vi "Elevator Controller.vi"(8 "error in (no error)":errorcluster, 9 "Notify when settled?":bool, 10 "State in":T2=enum."Tote 3", 11 "Elevator Inputs":T1={"Up"=FALSE, "Down"=FALSE, "Bin Modifier"=FALSE, "Pickup"=FALSE, "Top LS"=FALSE, "Bottom LS"=FALSE, "Encoder Position"=-2958.0, "Encoder Velocity"=0.0, "Manual Control"=-0.0}) -> (0 "error out":errorcluster, 1 "Settled?":bool=TRUE, 2 "Output":dbl=0.0975, 3 "State out":T2=enum."Tote 3")   [LabVIEW 2014]
uses:
  Elevator States.ctl
  Elevator Input Data.ctl
  Elevator Control Mode.ctl
  Utilities/Sensor Refname.ctl
  Elevator Direction.ctl
  <vilib>/Rock Robotics/Network Tables/SD Read Boolean.vi
  Robot Global Data.vi
  Utilities/Sensor Refname to String.vi
  <vilib>/Rock Robotics/Network Tables/SD Write Number.vi
  <vilib>/addons/control/pid/pid.llb/PID Advanced (DBL).vi
  <vilib>/addons/control/pid/NI_PID_pid.lvlib
panel:
  in  "Tab Control":enum32{"Inputs", "Outputs", "PID", "Config"}(tab)=enum."PID"
  in  "PID gains":T3={"proportional gain (Kc)"=-0.0025, "integral time (Ti, min)"=0.0, "derivative time (Td, min)"=0.0} {"derivative time (Td, min)" format="%.3f"; "integral time (Ti, min)" format="%.3f"; "proportional gain (Kc)" format="%.3f"}
  in  "PID output range":cluster{"output high":dbl, "output low":dbl}={"output high"=1.0, "output low"=-0.75} {"output low" format="%.2f"; "output high" format="%.2f"}
  in  "Setpoint range":cluster{"setpoint high":dbl, "setpoint low":dbl}={"setpoint high"=100.0, "setpoint low"=-6000.0} {"setpoint high" format="%.2f"; "setpoint low" format="%.2f"}
  in  "reinitialize? (F)":bool
  in  "Deadzone":dbl=0.15
  in  "Setpoint Diff":dbl=250.0
  in  "Motor Diff":dbl=2.0
  in  "Enable motor ramping?":bool
  in  "Enable setpoint chasing?":bool=TRUE
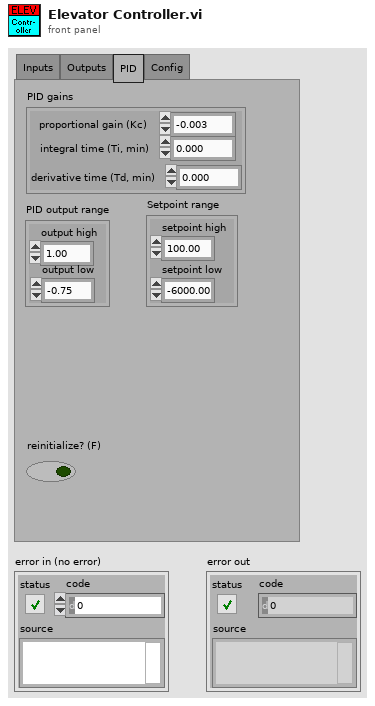
[diagram p1: front panel]
types:
  T1 = typedef "Elevator Input Data.ctl" = cluster{"Up":bool, "Down":bool, "Bin Modifier":bool, "Pickup":bool, "Top LS":bool, "Bottom LS":bool, "Encoder Position":dbl, "Encoder Velocity":dbl, "Manual Control":dbl}
  T2 = typedef "Elevator States.ctl" = enum16{"Ground", "Tote 1", "Tote 2", "Tote 3", "Tote 4", "Tote 5", "Tote 6"}
  T3 = cluster{"proportional gain (Kc)":dbl, "integral time (Ti, min)":dbl, "derivative time (Td, min)":dbl}
  T4 = typedef "Elevator Control Mode.ctl" = enum16{"PID", "PID to Manual", "Manual", "Manual to PID"}
  T5 = typedef "Sensor Refname.ctl" = enum16{"Gyro", "Elevator Top LS", "Elevator Bottom LS", "Claw Outside LS", "Left Drive Encoder", "Right Drive Encoder", "Strafe Encoder", "Elevator Encoder", "Ultrasonic Forward", "Ultrasonic Back", "Arm Angle POT", "Arm Clapper POT", "Accelerometer", "Tote LS", "DIP 1", "DIP 2", "DIP 3", "DIP 4"}
  T6 = typedef "Elevator Direction.ctl" = enum16{"Up", "Down"}
  T7 = typedef "WPI_PotentiometerDevRef.ctl" = cluster{"DevStatus":errorcluster, "Controller":T8, "Analog Channel":T9, "Invert Output":bool}
  T8 = typedef "FPGA_TypedefAnalogModule.ctl" = enum16{"Controller 1"}
  T9 = typedef "FPGA_AIChannel.ctl" = enum8{"AI 0", "AI 1", "AI 2", "AI 3", "AI MXP 0", "AI MXP 1", "AI MXP 2", "AI MXP 3", "Invalid"}
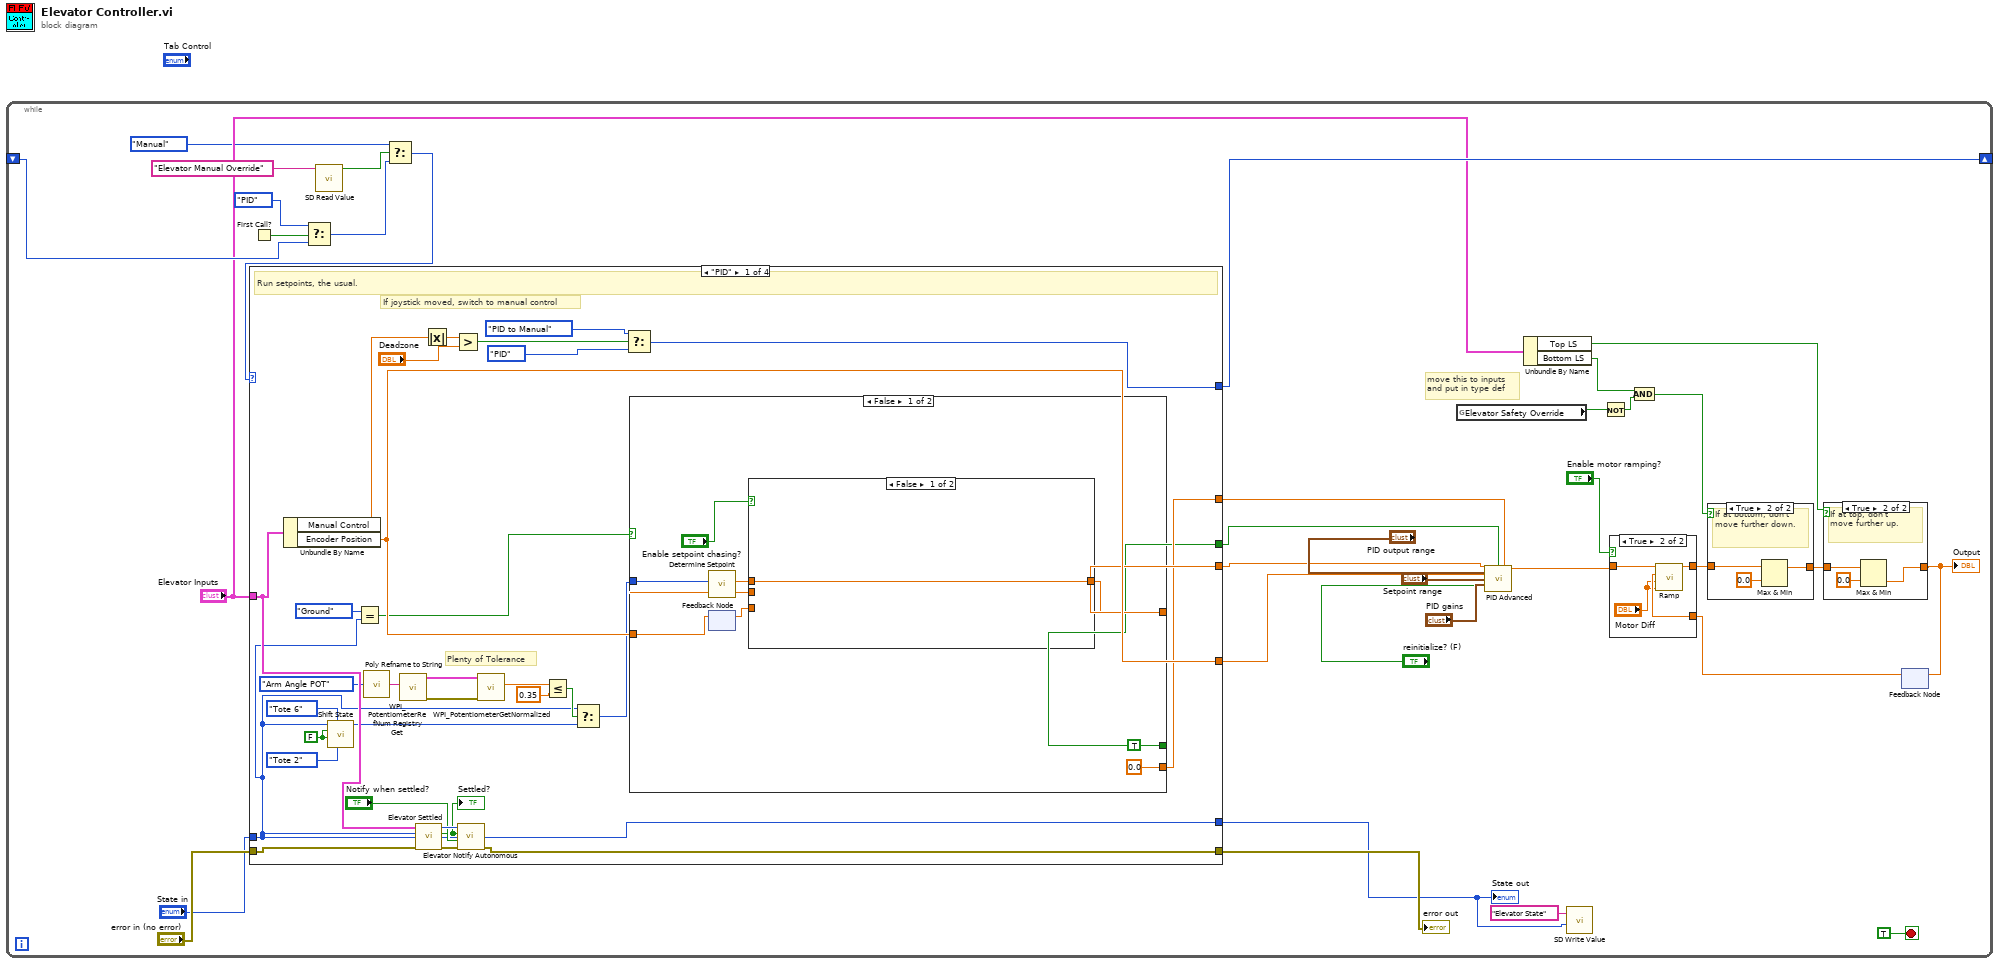
[diagram p0: block diagram]
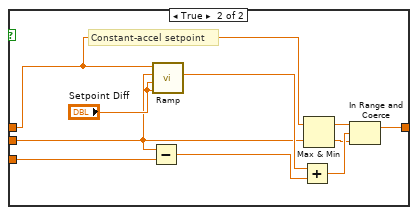
[diagram p5: hidden frame]
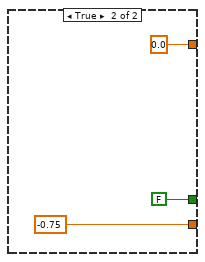
[diagram p6: hidden frame]
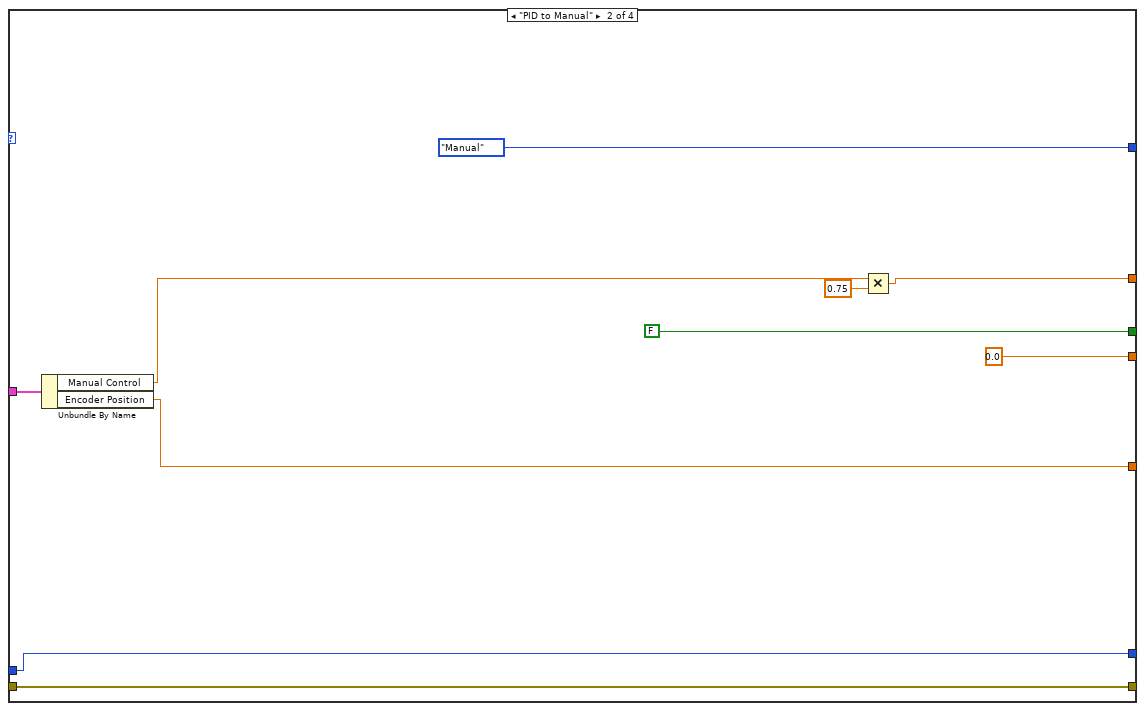
[diagram p7: hidden frame]
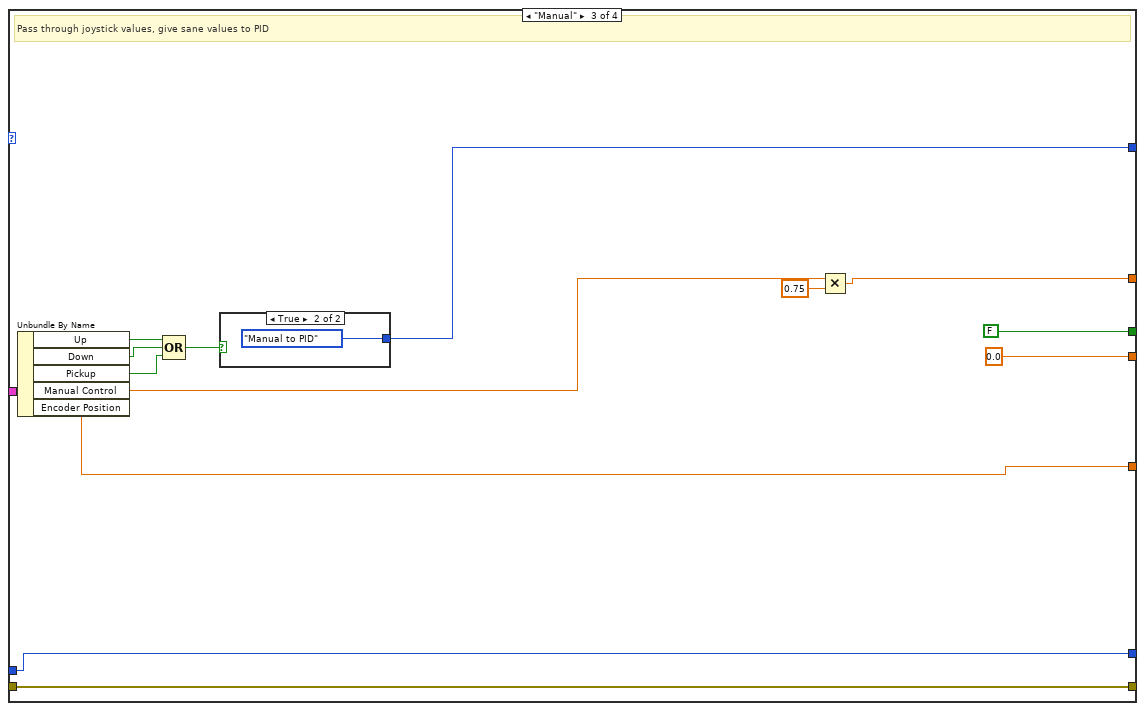
[diagram p8: hidden frame]
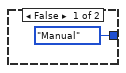
[diagram p9: hidden frame]
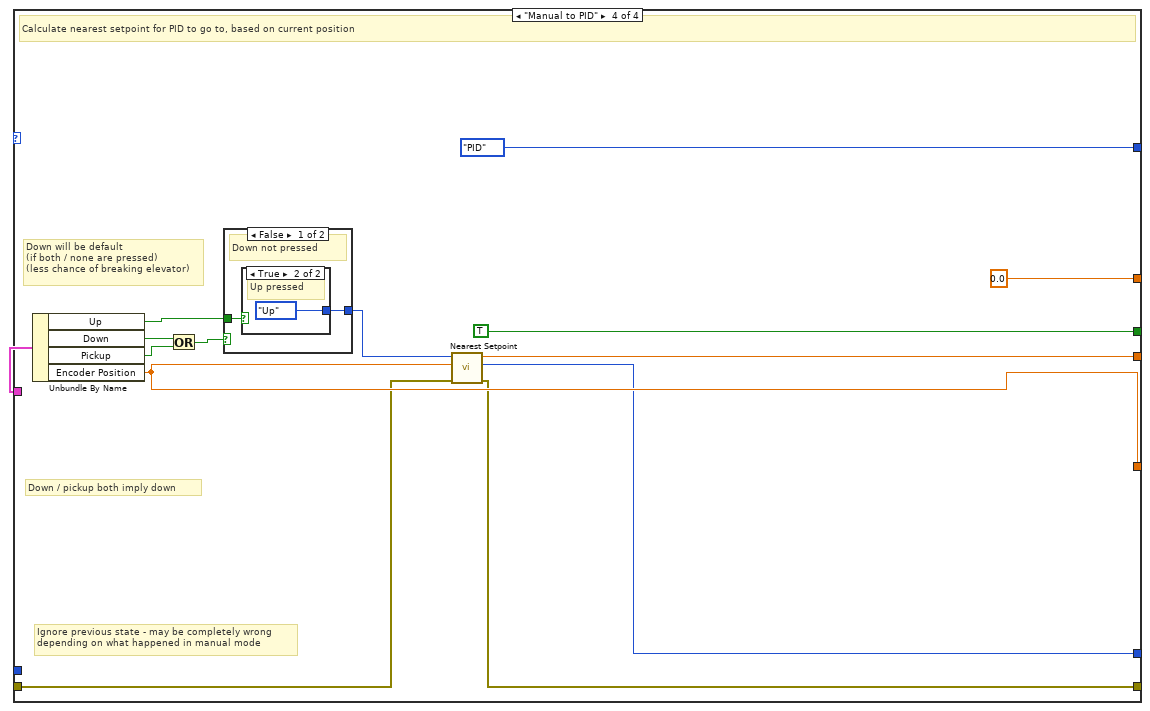
[diagram p10: hidden frame]
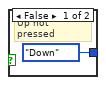
[diagram p11: hidden frame]
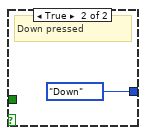
[diagram p12: hidden frame]
diagram:
  n1 = while {
    shift-right: [w33] -> _
    shift-left: _ -> [w35]
    stop <- TRUE stop-if-true
    # "move this to inputs \nand put in type def"
    n2 = First Call?() -> (First Call?: T/F=w5:bool)
    n3 = Select(t=Elevator_Control_Mode."PID", s=w5, f=w35) -> (s? t:f=w12:T4)
    n4 = call-poly <vilib>:"SD Read Value.vi"("Name"="Elevator Manual Override") -> ("Boolean"=w9:bool)  [unwired: 8 in, 2 out]
    n5 = Select(t=Elevator_Control_Mode."Manual", s=w9, f=w12) -> (s? t:f=w11:T4)
    n6 = case shown="\"PID\"" w11 {
      tunnel: "Elevator Inputs" -> [w77 w111 w127 w143]
      tunnel: [w66 0.0 ("Setpoint") 0.0 ("Manual Control") w137] -> w15
      tunnel: [w62 FALSE FALSE TRUE] -> w25
      tunnel: [w72 Elevator_Control_Mode."Manual" w121 Elevator_Control_Mode."PID"] -> w33
      tunnel: [w67 w110 w118 w134] -> w28
      tunnel: [w65 w105 w115 0.0 ("Manual Control")] -> w24
      tunnel: [w53 w107 w117 w132] -> w6
      tunnel: "State in" -> [w53 w107 w117 _]
      tunnel: "error in (no error)" -> [w71 w106 w116 w130]
      tunnel: [w70 w106 w116 w131] -> w21
      frame "PID" {
        w50 = FALSE
        # "Plenty of Tolerance"
        # "If joystick moved, switch to manual control"
        # "Run setpoints, the usual."
        n7 = Unbundle By Name(w77) -> ("Manual Control"=w74:dbl, "Encoder Position"=w67:dbl)
        n8 = call "Shift State.vi"("Lower bound"=Elevator_States."Tote 2" ("x"), "Upper bound"=Elevator_States."Tote 6" ("x"), "Decrement"=w50, "Increment"=w50, "State in"=w53) -> ("State out"=w49:i32)  [unwired: 6 in]
        n9 = Equal?(x=Elevator_States."Ground", y=w53) -> (x = y?=w64:bool)
        n10 = call-poly "Poly Refname to String.vi"("Sensor Refnames"=Sensor_Refname."Arm Angle POT" ("Sensor Refname")) -> ("Refname"=w60:string)
        n11 = call <vilib>:"WPI_PotentiometerRefNum Registry Get.vi"("refnum name"=w60) -> ("error out"=w58:errorcluster, "PotDevRef"=w59:T7)  [unwired: 9 in]
        n12 = call "Elevator Settled.vi"("error in (no error)"=w71, "State"=w53, "Elevator Inputs"=w77) -> ("error out"=w79:errorcluster, "Settled?"=w78:bool, "State"=w81:T2)  [unwired: 6 in]
        "Settled?" <- w78
        n13 = Absolute Value(x=w74) -> (abs(x)=w76:dbl)
        n14 = Greater?(x=w76, y="Deadzone") -> (0:w73:bool)
        n15 = call "Elevator Notify Autonomous.vi"("error in (no error)"=w79, "Notify when settled?"="Notify when settled?", "Settled?"=w78, "State"=w81) -> ("error out"=w70:errorcluster)  [unwired: 7 in]
        n16 = call <vilib>:"WPI_PotentiometerGetNormalized.vi"("error in"=w58, "PotDevRef"=w59) -> ("Normalized Value"=w57:dbl)  [unwired: 7 in, 2 out]
        n17 = Less Or Equal?(x=w57, y=0.35) -> (x <= y?=w55:bool)
        n18 = Select(t=w53, s=w55, f=w49) -> (s? t:f=w54:i32)
        n19 = Select(t=Elevator_Control_Mode."PID to Manual", s=w73, f=Elevator_Control_Mode."PID" ("t")) -> (s? t:f=w72:T4)
        n20 = case shown="False" w64 {
          tunnel: [TRUE FALSE] -> w62
          tunnel: w54 -> [w84 _]
          tunnel: [w87 0.0 ("Setpoint")] -> w66
          tunnel: w67 -> [w83 _]
          tunnel: [0.0 ("Manual Control") -0.75 ("Manual Control")] -> w65
          frame False {
            n21 = call "Determine Setpoint.vi"("Elevator State"=w84) -> ("Setpoint"=w85:dbl)  [unwired: 9 in, 1 out]
            n22 = feedback #1() -> (w82:dbl)  [unwired: 1 in]
            n23 = feedback-in #1(w83) -> ()
            n24 = case shown="False" "Enable setpoint chasing?" {
              tunnel: w85 -> [w90 w95]
              tunnel: [w90 w91] -> w87
              tunnel: w83 -> [_ w94]
              tunnel: w82 -> [_ w99]
              frame False {
              }
              frame True {
                # "Constant-accel setpoint"
                n25 = Subtract(x=w94, y=w99) -> (x-y=w97:dbl)
                n26 = call "Ramp.vi"("Negative Change"="Setpoint Diff", "Positive Change"="Setpoint Diff", "Prev Motor"=w94, "Input"=w95) -> ("Motor Output"=w100:dbl)  [unwired: 6 in, 1 out]
                n27 = Add(x=w100, y=w97) -> (x+y=w96:dbl)
                n28 = Max & Min(x=w95, y=w94) -> (max(x,y)=w93:dbl, min(x,y)=w92:dbl)
                n29 = In Range and Coerce(upper limit=w93, x=w96, lower limit=w92) -> (coerced(x)=w91:dbl)  [unwired: 1 out]
              }
            }
          }
          frame True {
          }
        }
      }
      frame "PID to Manual" {
        n30 = Unbundle By Name(w111) -> ("Manual Control"=w109:dbl, "Encoder Position"=w110:dbl)
        n31 = Multiply(x=w109, y=0.75) -> (x*y=w105:dbl)
      }
      frame "Manual" {
        # "Pass through joystick values, give sane values to PID"
        n32 = Unbundle By Name(w127) -> ("Up"=w125:bool, "Down"=w124:bool, "Pickup"=w123:bool, "Manual Control"=w120:dbl, "Encoder Position"=w118:dbl)
        n33 = Compound Arithmetic op=OR(w125, w124, w123) -> (w122:bool)
        n34 = case shown="True" w122 {
          tunnel: [Elevator_Control_Mode."Manual" Elevator_Control_Mode."Manual to PID"] -> w121
          frame False {
          }
          frame True {
          }
        }
        n35 = Multiply(x=w120, y=0.75) -> (x*y=w115:dbl)
      }
      frame "Manual to PID" {
        # "Ignore previous state - may be completely wrong\ndepending on what happened in manual mode"
        # "Down / pickup both imply down"
        # "Down will be default\n(if both / none are pressed)\n(less chance of breaking elevator)"
        # "Calculate nearest setpoint for PID to go to, based on current position"
        n36 = Unbundle By Name(w143) -> ("Up"=w139:bool, "Down"=w142:bool, "Pickup"=w141:bool, "Encoder Position"=w134:dbl)
        n37 = Or(x=w142, y=w141) -> (x .or. y?=w140:bool)
        n38 = case shown="False" w140 {
          tunnel: w139 -> [w144 _]
          tunnel: [w145 Elevator_Direction."Down" ("Direction")] -> w138
          frame False {
            # "Down not pressed"
            n39 = case shown="True" w144 {
              tunnel: [Elevator_Direction."Down" ("Direction") Elevator_Direction."Up" ("Direction")] -> w145
              frame False {
                # "Up not pressed"
              }
              frame True {
                # "Up pressed"
              }
            }
          }
          frame True {
            # "Down pressed"
          }
        }
        n40 = call "Nearest Setpoint.vi"("error in (no error)"=w130, "Encoder"=w134, "Direction"=w138) -> ("error out"=w131:errorcluster, "State"=w132:T2, "Setpoint"=w137:dbl)  [unwired: 6 in]
      }
    }
    "State out" <- w6
    "error out" <- w21
    n41 = global read "Robot Global Data.vi" "Elevator Safety Override"() -> (w2:bool)
    n42 = call-poly <vilib>:"PID Advanced.vi"("setpoint"=w15, "output range"="PID output range", "auto? (T)"=w25, "manual control"=w24, "process variable"=w28, "setpoint range"="Setpoint range", "PID gains"="PID gains", "reinitialize? (F)"="reinitialize? (F)") -> ("output"=w20:dbl)  [unwired: 6 in, 1 out]
    n43 = Unbundle By Name("Elevator Inputs") -> ("Top LS"=w31:bool, "Bottom LS"=w4:bool)
    n44 = call-poly <vilib>:"SD Write Value.vi"("Numeric"=w6, "Name"="Elevator State") -> ()  [unwired: 8 in, 2 out]
    n45 = Not(x=w2) -> (.not. x?=w3:bool)
    n46 = And(x=w4, y=w3) -> (x .and. y?=w1:bool)
    n47 = feedback #2() -> (w17:dbl)  [unwired: 1 in]
    n48 = case shown="True" "Enable motor ramping?" {
      tunnel: w20 -> [w36 w40]
      tunnel: [w36 w39] -> w19
      tunnel: w17 -> [_ w38]
      frame False {
      }
      frame True {
        n49 = call "Ramp.vi"("Negative Change"="Motor Diff", "Positive Change"="Motor Diff", "Prev Motor"=w38, "Input"=w40) -> ("Motor Output"=w39:dbl)  [unwired: 6 in, 1 out]
      }
    }
    n50 = case shown="True" w1 {
      tunnel: [w45 w48] -> w32
      tunnel: w19 -> [w45 w46]
      frame False {
      }
      frame True {
        # "If at bottom, don't move further down."
        n51 = Max & Min(x=w46, y=0.0 ("x")) -> (max(x,y)=w48:dbl)  [unwired: 1 out]
      }
    }
    n52 = case shown="True" w31 {
      tunnel: w32 -> [w41 w44]
      tunnel: [w41 w42] -> w18
      frame False {
      }
      frame True {
        # "If at top, don't\nmove further up."
        n53 = Max & Min(x=w44, y=0.0) -> (min(x,y)=w42:dbl)  [unwired: 1 out]
      }
    }
    "Output" <- w18
    n54 = feedback-in #2(w18) -> ()
  }
